vi "MSEncoder SubVI SignalRemarksAddNew.vi"(5 "Label":string, 7 "Scan time":dbl, 9 "mz 1":dbl, 10 "mz 0":dbl, 11 "MSEncoder in":refnum<class "MSEncoder.lvclass">) -> (2 "Len":u32, 3 "MSEncoder out":refnum<class "MSEncoder.lvclass">)   [LabVIEW 2018, in "MSEncoder.lvclass"]
uses:
  MSEncoder.lvclass
  MSEncoder.lvclass/MSEncoder.ctl
  PublicSubVI/Class/SigInfo/SigInfo.ctl
  PublicSubVI/Class/SigInfo/SigInfo.lvclass
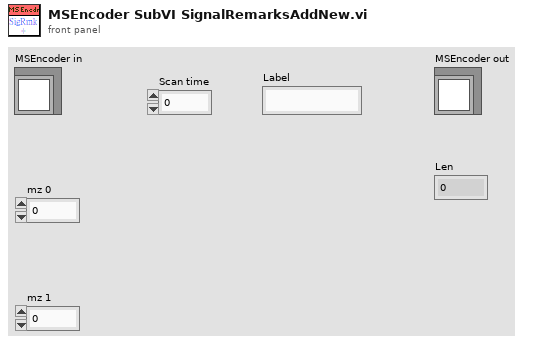
[diagram p1: front panel]
types:
  T1 = cluster{"Label":string, "dt":dbl, "Length":u32, "RefVolt":dbl, "mzTable":cluster{"t":dbl[], "mz":dbl[], "beta":dbl[]}}[]
  T2 = cluster{"Label":string, "dt":dbl, "Length":u32, "RefVolt":dbl, "mzTable":cluster{"t":dbl[], "mz":dbl[], "beta":dbl[]}}
  T3 = typedef "SigInfo.ctl" = enum16{"New mzList", "Set SigInfo", "Get SigInfo", "Append", "End"}
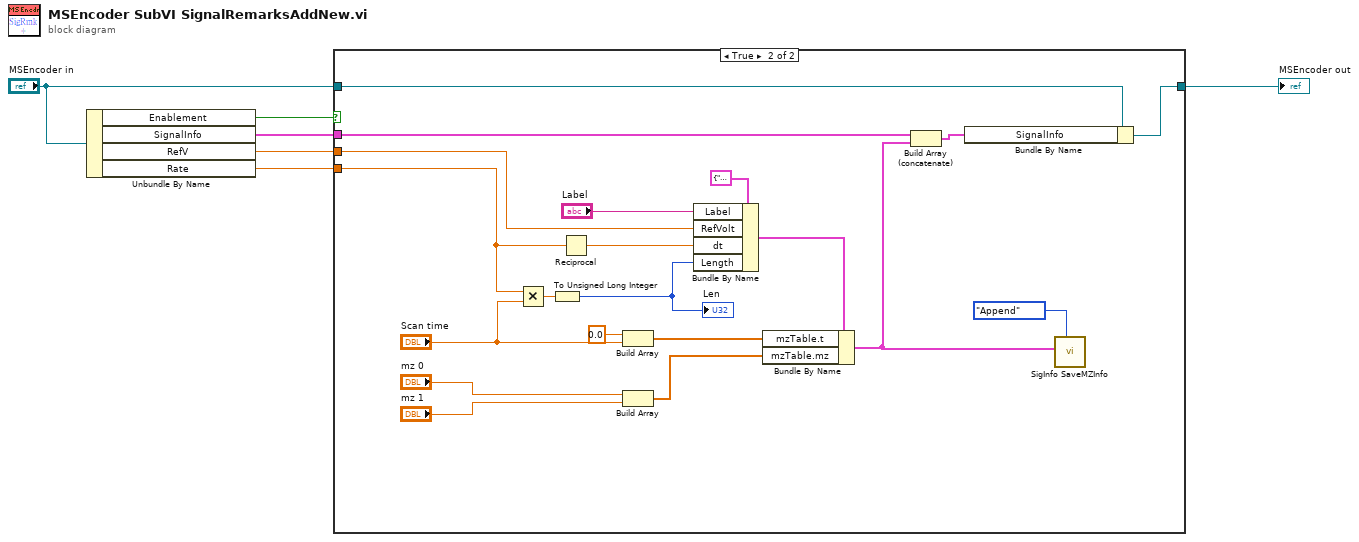
[diagram p0: block diagram]
diagram:
  n1 = Unbundle By Name("MSEncoder in") -> ("Enablement"=w1:bool, "SignalInfo"=w3:T1, "RefV"=w4:dbl, "Rate"=w6:dbl)
  n2 = case shown="True" w1 {
    tunnel: w6 -> [_ w27]
    tunnel: "MSEncoder in" -> [w7 w25]
    tunnel: w4 -> [_ w21]
    tunnel: w3 -> [_ w15]
    tunnel: [w7 w11] -> w2
    frame False {
    }
    frame True {
      n3 = Multiply(x=w27, y="Scan time") -> (x*y=w26:dbl)
      n4 = To Unsigned Long Integer(number=w26) -> (unsigned 32bit integer=w23:u32)
      "Len" <- w23
      n5 = Reciprocal(x=w27) -> (1/x=w24:dbl)
      n6 = Build Array(0.0 ("element"), "Scan time") -> (w12:dbl[])
      n7 = Build Array("mz 0", "mz 1") -> (w13:dbl[])
      n8 = Bundle By Name(cluster=T2 {"Label"="", "dt"=0.0, "Length"=0, "RefVolt"=0.0, "mzTable"={"t"=[], "mz"=[], "beta"=[]}} ("SigInfo"), "Label"="Label", "RefVolt"=w21, "dt"=w24, "Length"=w23) -> (w16:T2)
      n9 = Bundle By Name(cluster=w16, "mzTable.t"=w12, "mzTable.mz"=w13) -> (w8:T2)
      n10 = Build Array (concatenate)(w15, w8) -> (w14:T1)
      n11 = Bundle By Name(cluster=w25, "SignalInfo"=w14) -> (w11:refnum<class "MSEncoder.lvclass">)
      n12 = call "SigInfo SaveMZInfo.vi"("Function"=SigInfo."Append", "SigInfo"=w8) -> ()  [unwired: 7 in, 3 out]
    }
  }
  "MSEncoder out" <- w2
